vi "Create Channels.vi"(8 "error in (no error)":errorcluster, 10 "Default Channel Status":bool, 11 "Module Configuration in":refnum<class "Module Configuration.lvclass">) -> (0 "error out":errorcluster, 2 "All Channels[]":T1[](array[typedef]), 3 "Module Configuration out":refnum<class "Module Configuration.lvclass">)   [LabVIEW 2020, in "Plugin.lvlib" / "Plugin_UI.lvclass"]
doc: "Creates the Plugin Channel data."
uses:
  Plugin_UI.lvclass
  builds/Libraries/LabSys Framework.lvlibp/Configuration Storage/Module Configuration/Module Configuration.lvclass
  builds/Libraries/LabSys Framework.lvlibp/Configuration Storage/Test Configuration/Channel Information.ctl
  builds/Libraries/LabSys Framework.lvlibp/Configuration Storage/Test Configuration/Channel Directions.ctl
  builds/Libraries/LabSys Framework.lvlibp/Configuration Storage/Test Configuration/Scaling Information.ctl
  builds/Libraries/LabSys Framework.lvlibp/Configuration Storage/Test Configuration/Scaling Types.ctl
  builds/Libraries/Framework Base Library.lvlibp/Value Types.ctl
  builds/Libraries/LabSys Framework.lvlibp/Configuration Storage/Test Configuration/Subchannel Information.ctl
  Auxiliary Data.ctl
  Channels/Plugin_Channels.lvclass
  Channels/Input Channels/Input Channels.lvclass
  builds/Libraries/LabSys Framework.lvlibp/Configuration Storage/Test Configuration/Test Configuration.lvclass
  builds/Libraries/Framework Base Library.lvlibp
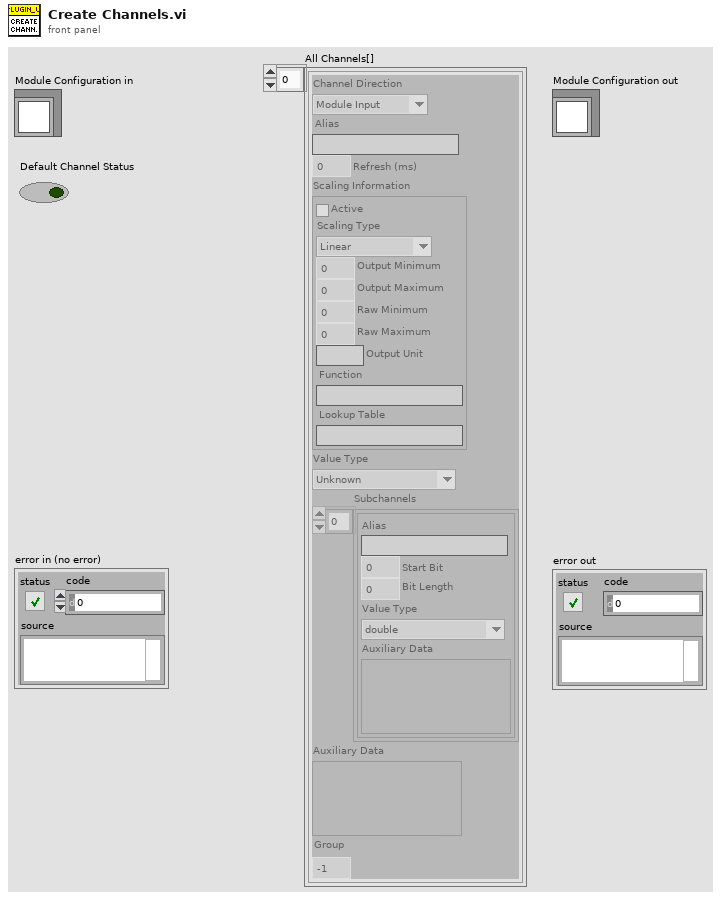
[diagram p1: front panel]
types:
  T1 = typedef "LabSys Framework.lvlibp/Configuration Storage.lvlib/Test Configuration.lvclass/Channel Information.ctl" = cluster{"Channel Direction":T2, "Alias":string, "Refresh (ms)":dbl, "Scaling Information":T3, "Value Type":T5, "Subchannels":T6[], "Auxiliary Data":variant, "Group":i32}
  T2 = typedef "LabSys Framework.lvlibp/Configuration Storage.lvlib/Test Configuration.lvclass/Channel Directions.ctl" = enum8{"Module Input", "Module Output"}
  T3 = typedef "LabSys Framework.lvlibp/Configuration Storage.lvlib/Test Configuration.lvclass/Scaling Information.ctl" = cluster{"Active":bool, "Scaling Type":T4, "Output Minimum":dbl, "Output Maximum":dbl, "Raw Minimum":dbl, "Raw Maximum":dbl, "Output Unit":string, "Function":string, "Lookup Table":string}
  T4 = typedef "LabSys Framework.lvlibp/Configuration Storage.lvlib/Test Configuration.lvclass/Scaling Types.ctl" = enum8{"Linear", "Function", "Lookup Table"}
  T5 = typedef "Framework Base Library.lvlibp/Value Types.ctl" = enum8{"Unknown", "double", "double array", "Waveform", "DigWaveform", "Boolean", "Decimal", "String", "Db2Message", "Byte Array", "Unsigned Decimal"}
  T6 = typedef "LabSys Framework.lvlibp/Configuration Storage.lvlib/Test Configuration.lvclass/Subchannel Information.ctl" = cluster{"Alias":string, "Start Bit":u32, "Bit Length":u32, "Value Type":T5, "Auxiliary Data":variant}
  T7 = typedef "Plugin.lvlib/Plugin_UI.lvclass/Auxiliary Data.ctl" = cluster{"Plugin_Data":refnum<class "Plugin_Channels.lvclass">}
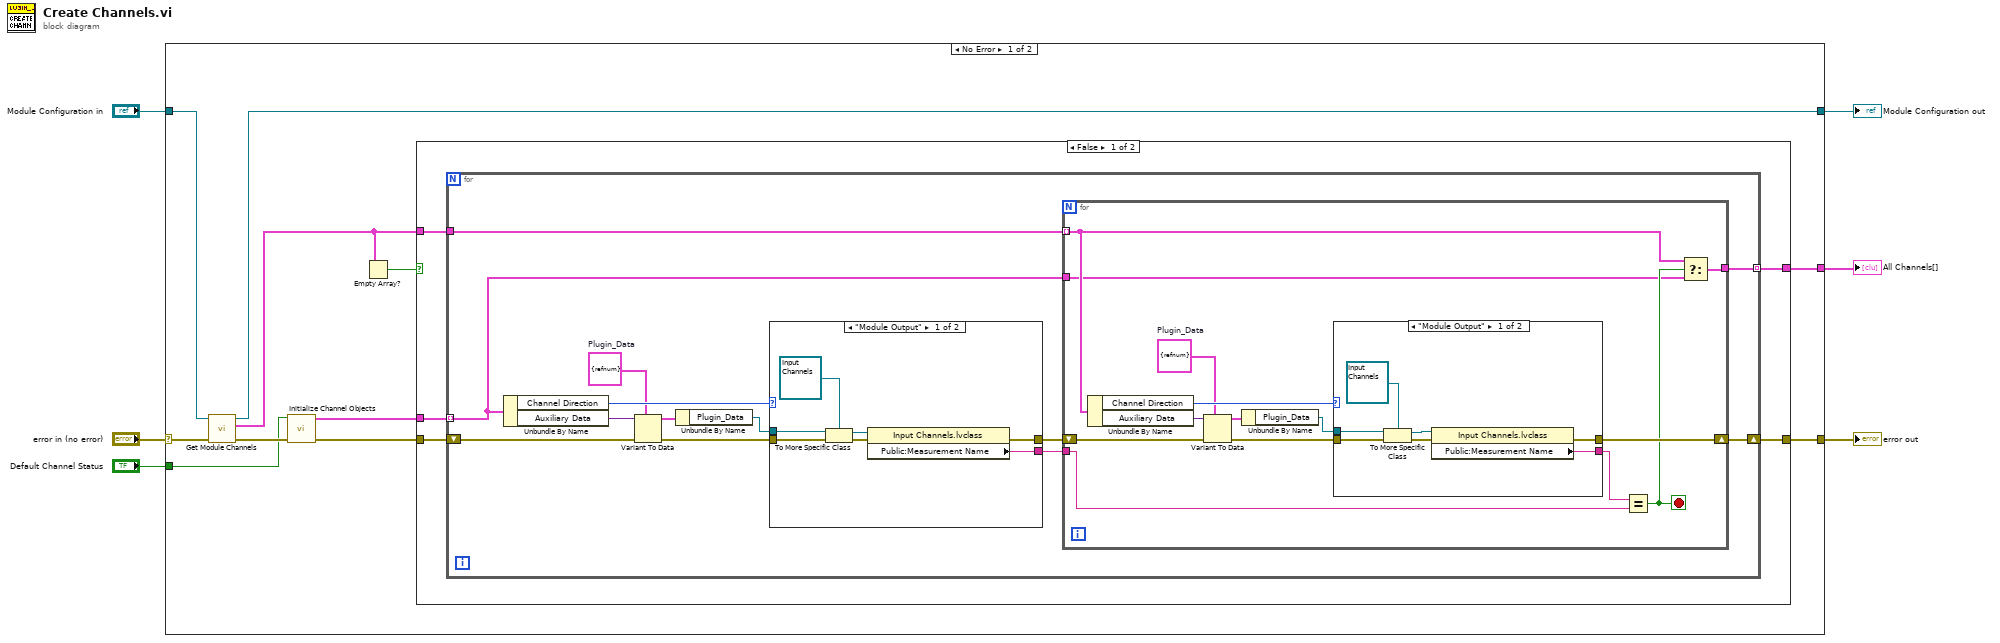
[diagram p0: block diagram]
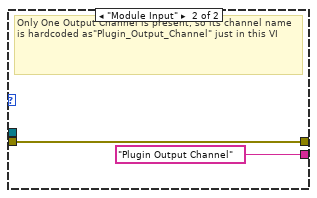
[diagram p2: hidden frame]
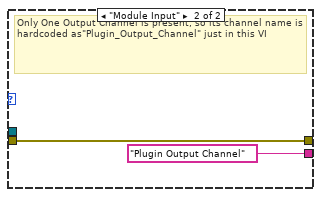
[diagram p3: hidden frame]
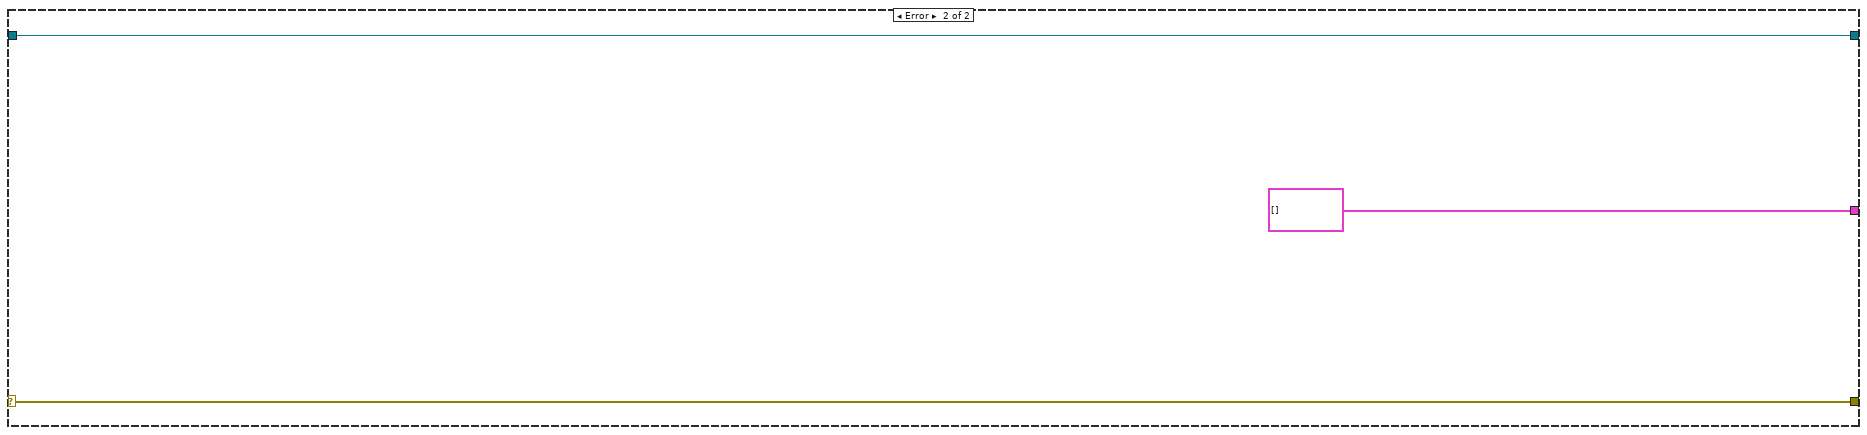
[diagram p5: hidden frame]
diagram:
  n1 = case shown="No Error" "error in (no error)" {
    selector: "error in (no error)" -> [w7 w72]
    tunnel: "Module Configuration in" -> [w17 w71]
    tunnel: [w16 w72] -> w5
    tunnel: [w15 T1[] [] ("Channel Info[]")] -> w4
    tunnel: [w14 w71] -> w3
    tunnel: "Default Channel Status" -> [w9 _]
    frame No Error {
      n2 = call-dynamic "Get Module Channels.vi"("error in (no error)"=w7, "Module Configuration in"=w17) -> ("error out"=w13:errorcluster, "Channel Information"=w10:T1[], "Module Configuration out"=w14:refnum<class "Module Configuration.lvclass">)  [unwired: 7 in]
      n3 = call "Initialize Channel Objects.vi"("error in (no error)"=w13, "Default Channel Status"=w9) -> ("error out"=w12:errorcluster, "Channel Info[]"=w11:T1[])  [unwired: 7 in, 1 out]
      n4 = Empty Array?(array=w10) -> (empty?=w8:bool)
      n5 = case shown="False" w8 {
        tunnel: w12 -> [w22 w68]
        tunnel: [w21 w68] -> w16
        tunnel: w10 -> [w18 _]
        tunnel: [w20 w69] -> w15
        tunnel: w11 -> [w19 w69]
        frame False {
          n6 = for {
            shift-right: [w29] -> w21
            shift-left: w22 -> [w35]
            tunnel: [w24] -> w20 mode=indexing
            tunnel: w19 -> [w25] mode=indexing
            tunnel: w18 -> [w23]
            w26 = T7 {"Plugin_Data"=refnum}  # Plugin_Data
            n7 = Unbundle By Name(w25) -> ("Channel Direction"=w27:T2, "Auxiliary Data"=w34:variant)
            n8 = Variant To Data(error in=w35, type=w26, Variant=w34) -> (data=w32:T7, error out=w33:errorcluster)
            n9 = Unbundle By Name(w32) -> ("Plugin_Data"=w31:refnum<class "Plugin_Channels.lvclass">)
            n10 = case shown="\"Module Output\"" w27 {
              tunnel: w33 -> [w65 w67]
              tunnel: w31 -> [w64 _]
              tunnel: [w61 w67] -> w30
              tunnel: [w60 "Plugin Output Channel" ("Public:Measurement Name")] -> w28
              frame "Module Output" {
                n11 = To More Specific Class(target class=refnum<class "Input Channels.lvclass"> refnum ("Plugin.lvlib:Input Channels.lvclass"), reference=w64, error in=w65) -> (specific class reference=w63:refnum<class "Input Channels.lvclass">, error out=w62:errorcluster)
                n12 = property class="Input Channels.lvclass"(reference=w63, error in=w62) -> (error out=w61:errorcluster, "Public:Measurement Name"=w60:string)  [unwired: 1 out]
              }
              frame "Module Input" {
                # "Only One Output Channel is present, so its channel name is hardcoded as\"Plugin_Output_Channel\" just in this VI"
              }
            }
            n13 = for {
              tunnel: w23 -> [w38] mode=indexing
              shift-right: [w43] -> w29
              shift-left: w30 -> [w44]
              tunnel: w28 -> [w41]
              tunnel: w25 -> [w37]
              tunnel: [w36] -> w24
              stop <- w39 stop-if-true
              w40 = T7 {"Plugin_Data"=refnum}  # Plugin_Data
              n14 = Unbundle By Name(w38) -> ("Channel Direction"=w45:T2, "Auxiliary Data"=w46:variant)
              n15 = Variant To Data(error in=w44, type=w40, Variant=w46) -> (data=w48:T7, error out=w47:errorcluster)
              n16 = Unbundle By Name(w48) -> ("Plugin_Data"=w49:refnum<class "Plugin_Channels.lvclass">)
              n17 = case shown="\"Module Output\"" w45 {
                tunnel: w47 -> [w56 w58]
                tunnel: w49 -> [w55 _]
                tunnel: [w52 w58] -> w43
                tunnel: [w51 "Plugin Output Channel" ("Public:Measurement Name")] -> w42
                frame "Module Output" {
                  n18 = To More Specific Class(target class=refnum<class "Input Channels.lvclass"> refnum ("Plugin.lvlib:Input Channels.lvclass"), reference=w55, error in=w56) -> (specific class reference=w54:refnum<class "Input Channels.lvclass">, error out=w53:errorcluster)
                  n19 = property class="Input Channels.lvclass"(reference=w54, error in=w53) -> (error out=w52:errorcluster, "Public:Measurement Name"=w51:string)  [unwired: 1 out]
                }
                frame "Module Input" {
                  # "Only One Output Channel is present, so its channel name is hardcoded as\"Plugin_Output_Channel\" just in this VI"
                }
              }
              n20 = Equal?(x=w42, y=w41) -> (x = y?=w39:bool)
              n21 = Select(t=w38, s=w39, f=w37) -> (s? t:f=w36:T1)
            }
          }
        }
        frame True {
        }
      }
    }
    frame Error {
    }
  }
  "error out" <- w5
  "All Channels[]" <- w4
  "Module Configuration out" <- w3
